vi "Button_Detect.vi"(10 "Input Cluster":T1={"Level 5"=TRUE, "Level 4"=TRUE, "Level 3"=TRUE, "Level 2"=TRUE, "Level 1"=FALSE}) -> (2 "Output Cluster":T1)   [LabVIEW 2014]
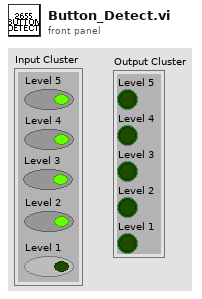
[diagram p1: front panel]
types:
  T1 = cluster{"Level 5":bool, "Level 4":bool, "Level 3":bool, "Level 2":bool, "Level 1":bool}
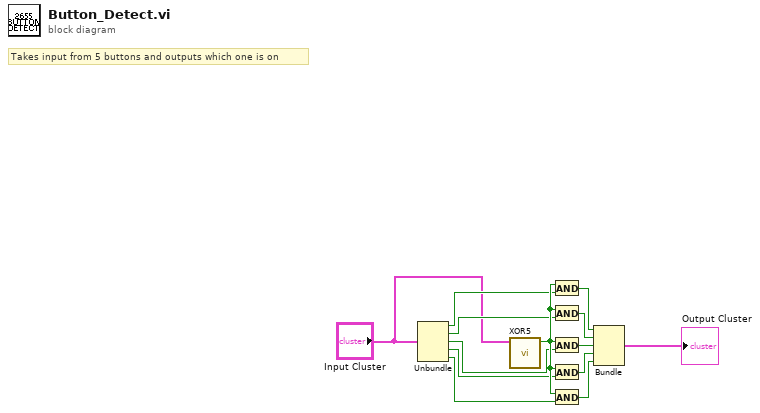
[diagram p0: block diagram]
diagram:
  # "Takes input from 5 buttons and outputs which one is on"
  n1 = Unbundle("Input Cluster") -> ("Level 5"=w12:bool, "Level 4"=w11:bool, "Level 3"=w8:bool, "Level 2"=w9:bool, "Level 1"=w10:bool)
  n2 = call "XOR5.vi"("inputs"="Input Cluster") -> ("XOR5"=w13:bool)  [unwired: 10 in]
  n3 = And(x=w13, y=w12) -> (x .and. y?=w7:bool)
  n4 = And(x=w13, y=w11) -> (x .and. y?=w6:bool)
  n5 = And(x=w13, y=w8) -> (x .and. y?=w5:bool)
  n6 = And(x=w13, y=w9) -> (x .and. y?=w4:bool)
  n7 = And(x=w13, y=w10) -> (x .and. y?=w3:bool)
  n8 = Bundle(w7, w6, w5, w4, w3) -> (→"Output Cluster":cluster{bool, bool, bool, bool, bool})  [unwired: 1 in]
